vi "lockin - replace AO DC.vi"(8 "error in (no error)":errorcluster, 10 "AO.DC (V)":dbl[](array[numeric]), 11 "LockinDAQ":refnum<class "LockinDAQ.lvclass">) -> (0 "error out":errorcluster, 3 "LockinDAQ out":refnum<class "LockinDAQ.lvclass">)   [LabVIEW 2016, in "LockinDAQ.lvclass"]
uses:
  LockinDAQ.lvclass
  LockinDAQ.lvclass/LockinDAQ.ctl
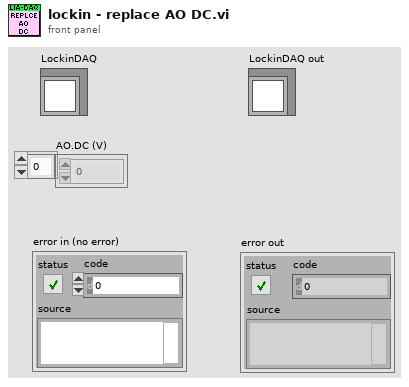
[diagram p1: front panel]
types:
  T1 = typedef "LockinDAQ.lvclass/AO-cluster.ctl" = cluster{"Ch":i32[], "Amp (V)":dbl[], "DC (V)":dbl[], "f (Hz)":dbl[], "Phase (°)":dbl[], "Function":T2[], "Sweep?":bool[]}
  T2 = typedef "LockinDAQ.lvclass/Function-enum.ctl" = enum16{"Sine", "Triangle", "Square", "Sawtooth"}
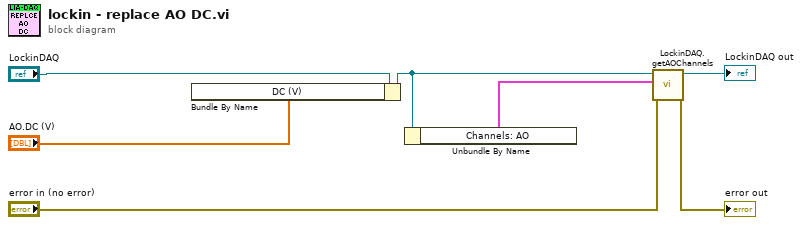
[diagram p0: block diagram]
diagram:
  n1 = Bundle By Name(cluster="LockinDAQ", "DC (V)"="AO.DC (V)") -> (w4:refnum<class "LockinDAQ.lvclass">)
  n2 = Unbundle By Name(w4) -> ("Channels: AO"=w5:T1)
  n3 = call "LockinDAQ.getAOChannels.vi"("error in (no error)"="error in (no error)", "Channels: AO"=w5, "LockinDAQ"=w4) -> ("error out"=→"error out":errorcluster, "LockinDAQ out"=→"LockinDAQ out":refnum<class "LockinDAQ.lvclass">)  [unwired: 7 in]
